vi "singin.vi"(0 "sim I/O info in":T1, 9 "data from node input terminals":variant[](array[variant]), 11 "input from node terminal error in":errorcluster) -> (4 "sim I/O info out":T1, 10 "data to node output terminals":variant[](array[variant]), 15 "output to node terminal error out":errorcluster)   [LabVIEW 2012]
uses:
  <vilib>/FPGA/viExecutionOnDevComputer/simIO/customVI/Sim IO Info.ctl
  <vilib>/rvi/customViForEmulation/niLvFPGAUserSpecifiedEmulationVISupport.lvclass
  <vilib>/FPGA/viExecutionOnDevComputer/simIO/customVI/niFPGA Simulated IO.lvlib
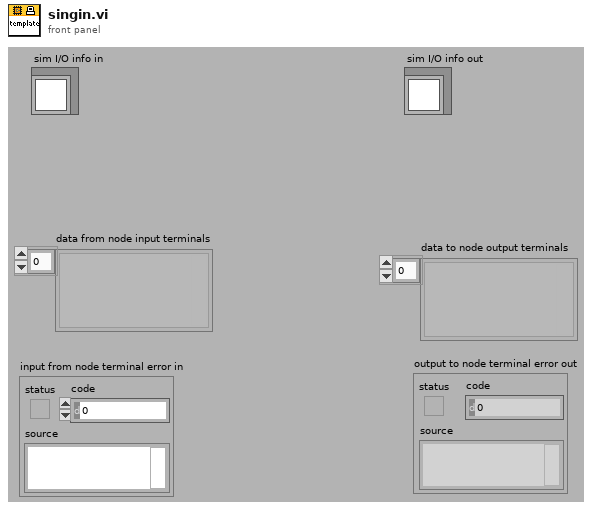
[diagram p1: front panel]
types:
  T1 = typedef "niFPGA Simulated IO.lvlib/Sim IO Info.ctl" = refnum<class "niLvFPGAUserSpecifiedEmulationVISupport.lvclass">
  T2 = typedef "niFPGA Simulated IO.lvlib/Execution Stage.ctl" = enum16{"Initializing", "Running", "Shutting Down"}
  T3 = typedef "niFPGA Simulated IO.lvlib/Node or Element Type.ctl" = enum16{"Read I/O", "Write I/O", "Method", "Read Property", "Write Property"}
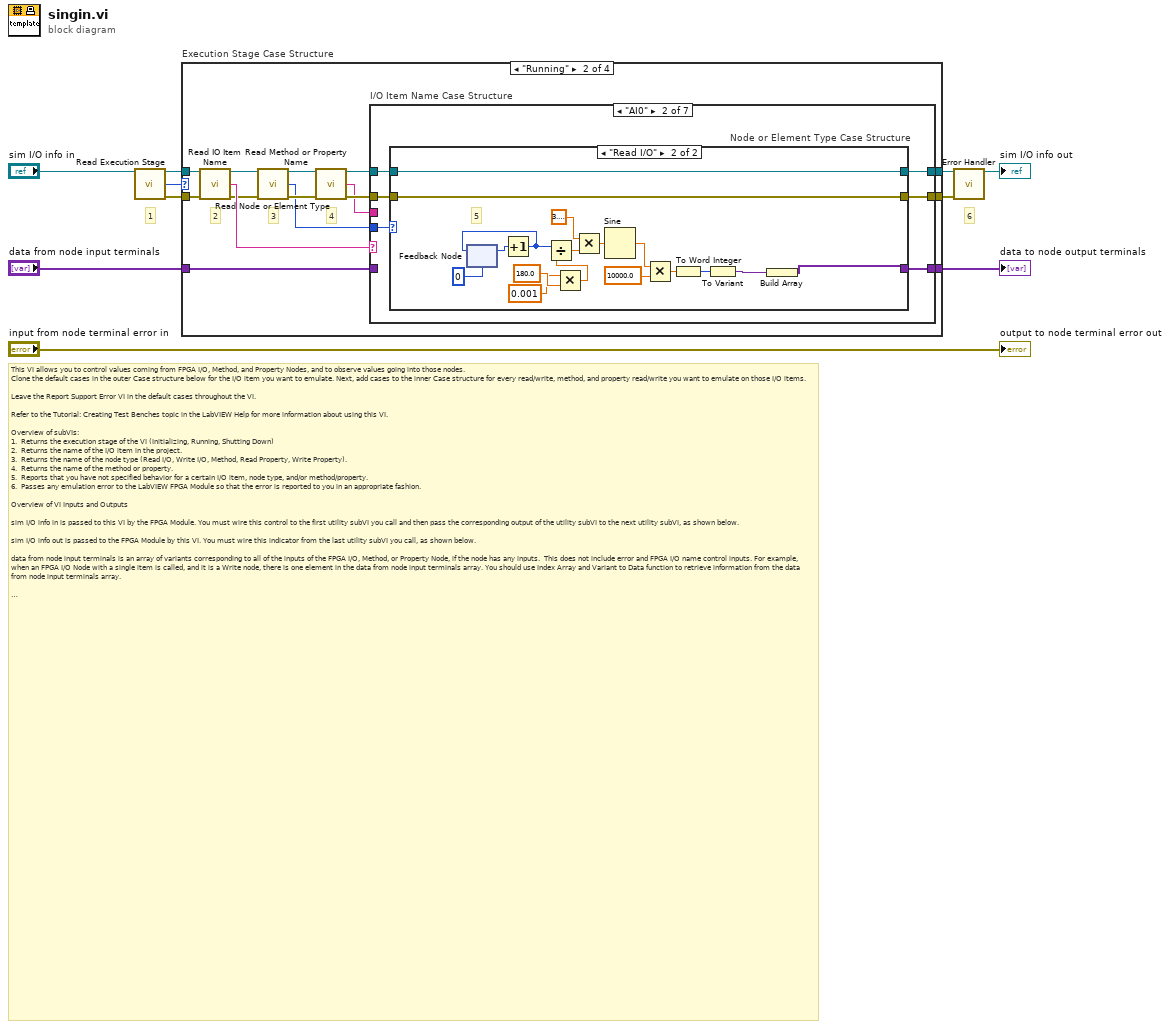
[diagram p0: block diagram]
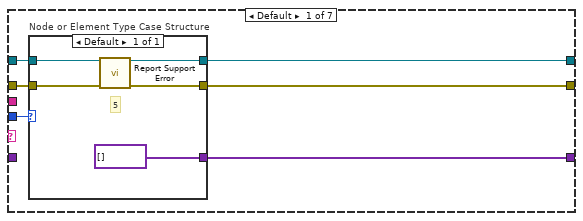
[diagram p3: hidden frame]
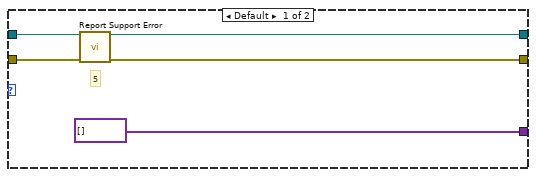
[diagram p4: hidden frame]
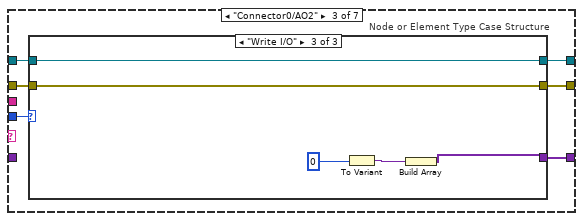
[diagram p5: hidden frame]
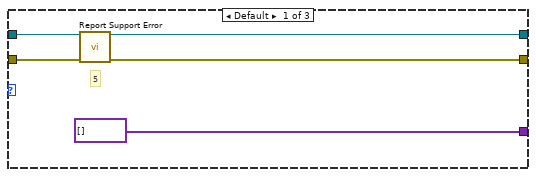
[diagram p6: hidden frame]
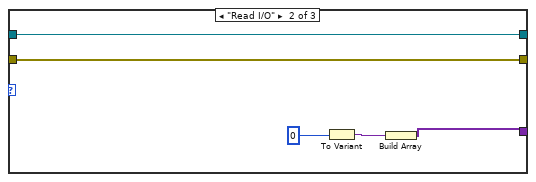
[diagram p7: hidden frame]
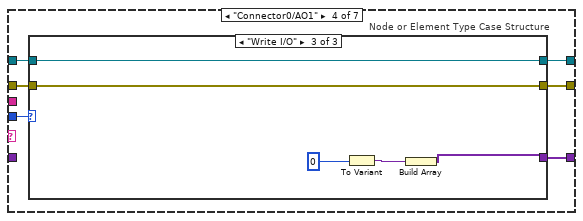
[diagram p8: hidden frame]
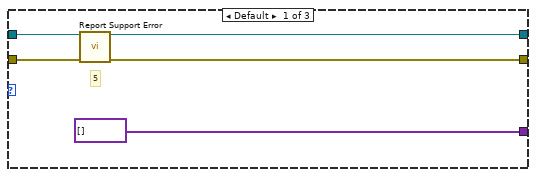
[diagram p9: hidden frame]
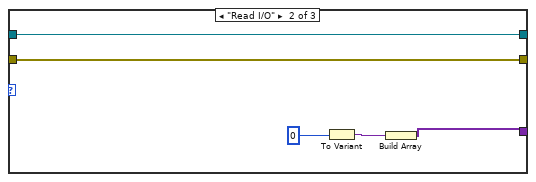
[diagram p10: hidden frame]
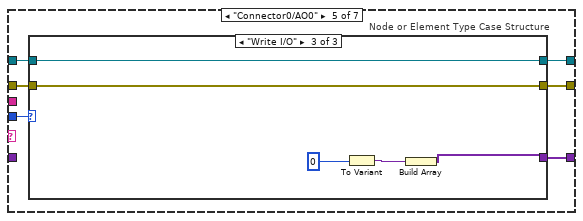
[diagram p11: hidden frame]
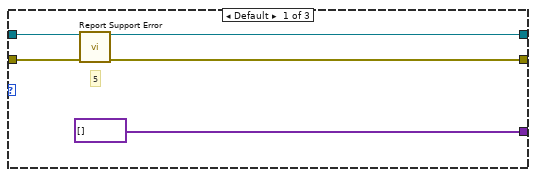
[diagram p12: hidden frame]
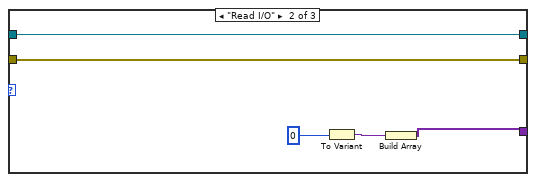
[diagram p13: hidden frame]
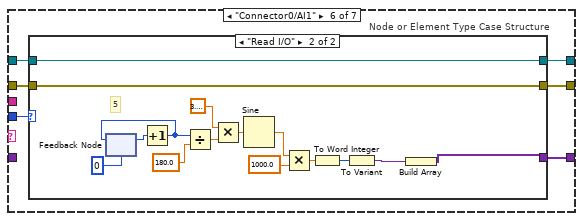
[diagram p14: hidden frame]
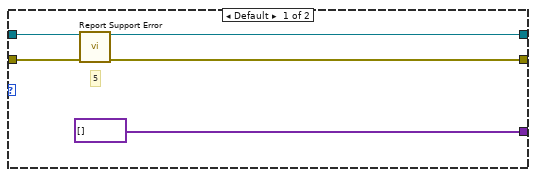
[diagram p15: hidden frame]
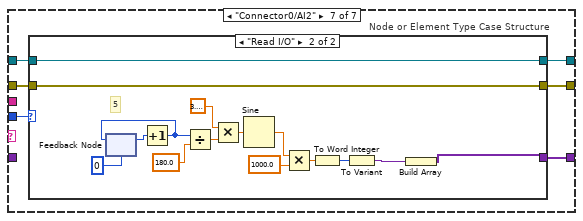
[diagram p16: hidden frame]
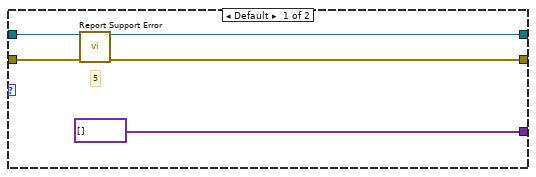
[diagram p17: hidden frame]
diagram:
  # "1"
  # "6"
  # "This VI allows you to control values coming from FPGA I/O, Method, and Property Nodes, and to observe values going into those nodes.\nClone the default cases in the outer Case structure below for the I/O item you want to emulate. Next, add cases to the inner Case structure for every read/write, method, and property read/write you want to emulate on those I/O items.  \n\nLeave the Report Support Error VI in the default cases throughout the VI.\n\nRefer to the Tutorial: Creating Test Benches topic in the LabVIEW Help for more information about using this VI.\n\nOverview of subVIs:\n1.  Returns the execution stage of the VI (Initializing, Running, Shutting Down)\n2.  Returns the name of the I/O item in the project.\n3.  Returns the name of the node type (Read I/O, Write I/O, Method, Read Property, Write Property).\n4.  Returns the name of the method or property.\n5.  Reports that you have not specified behavior for a certain I/O item, node type, and/or method/property.\n6.  Passes any emulation error to the LabVIEW FPGA Module so that the error is reported to you in an appropriate fashion.\n\nOverview of VI Inputs and Outputs\n\nsim I/O info in is passed to this VI by the FPGA Module. You must wire this control to the first utility subVI you call and then pass the corresponding output of the utility subVI to the next utility subVI, as shown below.\n\nsim I/O info out is passed to the FPGA Module by this VI. You must wire this indicator from the last utility subVI you call, as shown below.\n\ndata from node input terminals is an array of variants corresponding to all of the inputs of the FPGA I/O, Method, or Property Node, if the node has any inputs.  This does not include error and FPGA I/O name control inputs. For example, when an FPGA I/O Node with a single item is called, and it is a Write node, there is one element in the data from node input terminals array. You should use Index Array and Variant to Data function to retrieve information from the data from node input terminals array.\n\ndata to node output terminals is an array of variants corresponding to all the outputs of the FPGA I/O, Method, or Property Node, if the node has any outputs.  This does not include error and FPGA I/O name control outputs. For example, when an FPGA I/O node with a single item is called, and it is a Read node, there should be one element in the data to node output terminals array. You should use To Variant and Build Array functions to pass the information to the data to node output terminals array.\n\ninput from node terminal error in is the error that gets passed into the FPGA I/O, Method, or Property Node, if the node is configured so that the error input is shown. If the node is configured so that the error input is not shown, the value of this input corresponds to \"no error\" (status is false, error code is 0). \n\noutput to node terminal error out is the error that gets passed out of the FPGA I/O, Method, or Property Node, if the node is configured so that the error output is shown.  If the node is configured so that the error output is not shown, the value of this output is ignored."
  n1 = call <vilib>:"Read Execution Stage.vi"("sim I/O info in"="sim I/O info in") -> ("sim I/O info out"=w3:T1, "execution stage"=w1:T2, "error out"=w2:errorcluster)  [unwired: 1 in, 11 out]
  n2 = case "Execution Stage Case Structure" shown="\"Running\"" w1 {
    tunnel: [_ w26 _ _] -> w9
    tunnel: [w12 w21 w183 w185] -> w4
    tunnel: [w11 w17 w182 w184] -> w6
    tunnel: w3 -> [w11 w15 w182 w184]
    tunnel: w2 -> [w12 w14 w183 w185]
    tunnel: "data from node input terminals" -> [_ w27 _ _]
    frame "Initializing" {
    }
    frame "Running" {
      # "4"
      # "3"
      # "2"
      n3 = call <vilib>:"Read IO Item Name.vi"("sim I/O info in"=w15, "error in (no error)"=w14) -> ("sim I/O info out"=w16:T1, "I/O item name"=w25:string, "error out"=w24:errorcluster)  [unwired: 11 out]
      n4 = call <vilib>:"Read Node or Element Type.vi"("sim I/O info in"=w16, "error in (no error)"=w24) -> ("sim I/O info out"=w13:T1, "node or element type"=w22:T3, "error out"=w23:errorcluster)  [unwired: 11 out]
      n5 = call <vilib>:"Read Method or Property Name.vi"("sim I/O info in"=w13, "error in (no error)"=w23) -> ("sim I/O info out"=w19:T1, "method or property name"=w18:string, "error out"=w20:errorcluster)  [unwired: 11 out]
      n6 = case "I/O Item Name Case Structure" shown="\"AI0\"" w25 {
        tunnel: w27 -> [_ _ _ _ _ _ _]
        tunnel: [w29 w40 w68 w89 w110 w131 w157] -> w26
        tunnel: w20 -> [w33 w44 w72 w93 w114 w135 w161]
        tunnel: [w32 w43 w71 w92 w113 w134 w160] -> w21
        tunnel: w19 -> [w31 w42 w70 w91 w112 w133 w159]
        tunnel: [w30 w41 w69 w90 w111 w132 w158] -> w17
        tunnel: w22 -> [w28 w39 w67 w88 w109 w130 w156]
        tunnel: w18 -> [_ _ _ _ _ _ _]
        frame Default {
          n7 = case "Node or Element Type Case Structure" shown="Default" w28 {
            tunnel: w33 -> [w38]
            tunnel: [w37] -> w32
            tunnel: w31 -> [w36]
            tunnel: [w35] -> w30
            tunnel: [variant[] []] -> w29
            frame Default {
              # "5"
              n8 = call <vilib>:"Report Support Error.vi"("sim I/O info in"=w36, "error in (no error)"=w38) -> ("sim I/O info out"=w35:T1, "error out"=w37:errorcluster)  [unwired: 12 out]
            }
          }
        }
        frame "AI0" {
          n9 = case "Node or Element Type Case Structure" shown="\"Read I/O\"" w39 {
            tunnel: w44 -> [w49 w65]
            tunnel: [w48 w65] -> w43
            tunnel: w42 -> [w47 w66]
            tunnel: [w46 w66] -> w41
            tunnel: [variant[] [] w55] -> w40
            frame Default {
              # "5"
              n10 = call <vilib>:"Report Support Error.vi"("sim I/O info in"=w47, "error in (no error)"=w49) -> ("sim I/O info out"=w46:T1, "error out"=w48:errorcluster)  [unwired: 12 out]
            }
            frame "Read I/O" {
              # "5"
              n11 = feedback #1(0) -> (w57:i32)
              n12 = Increment(x=w57) -> (x+1=w56:i32)
              n13 = feedback-in #1(w56) -> ()
              n14 = Multiply(x=0.001, y=180.0) -> (x*y=w50:dbl)
              n15 = Divide(x=w56, y=w50) -> (x/y=w59:dbl)
              n16 = Multiply(x=3.141592653589793, y=w59) -> (x*y=w61:dbl)
              n17 = Sine(x=w61) -> (sin(x)=w63:dbl)
              n18 = Multiply(x=w63, y=10000.0) -> (x*y=w64:dbl)
              n19 = To Word Integer(number=w64) -> (16bit integer=w54:i16)
              n20 = To Variant(anything=w54) -> (Variant=w53:variant)
              n21 = Build Array(w53) -> (w55:variant[])
            }
          }
        }
        frame "Connector0/AO2" {
          n22 = case "Node or Element Type Case Structure" shown="\"Write I/O\"" w67 {
            tunnel: w72 -> [w77 w81 w86]
            tunnel: [w76 w81 w86] -> w71
            tunnel: w70 -> [w75 w82 w87]
            tunnel: [w74 w82 w87] -> w69
            tunnel: [variant[] [] w80 w85] -> w68
            frame Default {
              # "5"
              n23 = call <vilib>:"Report Support Error.vi"("sim I/O info in"=w75, "error in (no error)"=w77) -> ("sim I/O info out"=w74:T1, "error out"=w76:errorcluster)  [unwired: 12 out]
            }
            frame "Read I/O" {
              n24 = To Variant(anything=0) -> (Variant=w79:variant)
              n25 = Build Array(w79) -> (w80:variant[])
            }
            frame "Write I/O" {
              n26 = To Variant(anything=0) -> (Variant=w84:variant)
              n27 = Build Array(w84) -> (w85:variant[])
            }
          }
        }
        frame "Connector0/AO1" {
          n28 = case "Node or Element Type Case Structure" shown="\"Write I/O\"" w88 {
            tunnel: w93 -> [w98 w102 w107]
            tunnel: [w97 w102 w107] -> w92
            tunnel: w91 -> [w96 w103 w108]
            tunnel: [w95 w103 w108] -> w90
            tunnel: [variant[] [] w101 w106] -> w89
            frame Default {
              # "5"
              n29 = call <vilib>:"Report Support Error.vi"("sim I/O info in"=w96, "error in (no error)"=w98) -> ("sim I/O info out"=w95:T1, "error out"=w97:errorcluster)  [unwired: 12 out]
            }
            frame "Read I/O" {
              n30 = To Variant(anything=0) -> (Variant=w100:variant)
              n31 = Build Array(w100) -> (w101:variant[])
            }
            frame "Write I/O" {
              n32 = To Variant(anything=0) -> (Variant=w105:variant)
              n33 = Build Array(w105) -> (w106:variant[])
            }
          }
        }
        frame "Connector0/AO0" {
          n34 = case "Node or Element Type Case Structure" shown="\"Write I/O\"" w109 {
            tunnel: w114 -> [w119 w123 w128]
            tunnel: [w118 w123 w128] -> w113
            tunnel: w112 -> [w117 w124 w129]
            tunnel: [w116 w124 w129] -> w111
            tunnel: [variant[] [] w122 w127] -> w110
            frame Default {
              # "5"
              n35 = call <vilib>:"Report Support Error.vi"("sim I/O info in"=w117, "error in (no error)"=w119) -> ("sim I/O info out"=w116:T1, "error out"=w118:errorcluster)  [unwired: 12 out]
            }
            frame "Read I/O" {
              n36 = To Variant(anything=0) -> (Variant=w121:variant)
              n37 = Build Array(w121) -> (w122:variant[])
            }
            frame "Write I/O" {
              n38 = To Variant(anything=0) -> (Variant=w126:variant)
              n39 = Build Array(w126) -> (w127:variant[])
            }
          }
        }
        frame "Connector0/AI1" {
          n40 = case "Node or Element Type Case Structure" shown="\"Read I/O\"" w130 {
            tunnel: w135 -> [w140 w154]
            tunnel: [w139 w154] -> w134
            tunnel: w133 -> [w138 w155]
            tunnel: [w137 w155] -> w132
            tunnel: [variant[] [] w143] -> w131
            frame Default {
              # "5"
              n41 = call <vilib>:"Report Support Error.vi"("sim I/O info in"=w138, "error in (no error)"=w140) -> ("sim I/O info out"=w137:T1, "error out"=w139:errorcluster)  [unwired: 12 out]
            }
            frame "Read I/O" {
              # "5"
              n42 = feedback #2(0) -> (w145:i32)
              n43 = Increment(x=w145) -> (x+1=w144:i32)
              n44 = feedback-in #2(w144) -> ()
              n45 = Divide(x=w144, y=180.0) -> (x/y=w148:dbl)
              n46 = Multiply(x=3.141592653589793, y=w148) -> (x*y=w150:dbl)
              n47 = Sine(x=w150) -> (sin(x)=w152:dbl)
              n48 = Multiply(x=w152, y=1000.0) -> (x*y=w153:dbl)
              n49 = To Word Integer(number=w153) -> (16bit integer=w142:i16)
              n50 = To Variant(anything=w142) -> (Variant=w141:variant)
              n51 = Build Array(w141) -> (w143:variant[])
            }
          }
        }
        frame "Connector0/AI2" {
          n52 = case "Node or Element Type Case Structure" shown="\"Read I/O\"" w156 {
            tunnel: w161 -> [w166 w180]
            tunnel: [w165 w180] -> w160
            tunnel: w159 -> [w164 w181]
            tunnel: [w163 w181] -> w158
            tunnel: [variant[] [] w169] -> w157
            frame Default {
              # "5"
              n53 = call <vilib>:"Report Support Error.vi"("sim I/O info in"=w164, "error in (no error)"=w166) -> ("sim I/O info out"=w163:T1, "error out"=w165:errorcluster)  [unwired: 12 out]
            }
            frame "Read I/O" {
              # "5"
              n54 = feedback #3(0) -> (w171:i32)
              n55 = Increment(x=w171) -> (x+1=w170:i32)
              n56 = feedback-in #3(w170) -> ()
              n57 = Divide(x=w170, y=180.0) -> (x/y=w174:dbl)
              n58 = Multiply(x=3.141592653589793, y=w174) -> (x*y=w176:dbl)
              n59 = Sine(x=w176) -> (sin(x)=w178:dbl)
              n60 = Multiply(x=w178, y=1000.0) -> (x*y=w179:dbl)
              n61 = To Word Integer(number=w179) -> (16bit integer=w168:i16)
              n62 = To Variant(anything=w168) -> (Variant=w167:variant)
              n63 = Build Array(w167) -> (w169:variant[])
            }
          }
        }
      }
    }
    frame "Shutting Down" {
    }
    frame Default {
    }
  }
  "data to node output terminals" <- w9
  n64 = call <vilib>:"Error Handler.vi"("sim I/O info in"=w6, "error in"=w4) -> ("sim I/O info out"=→"sim I/O info out":T1)  [unwired: 13 out]
  "output to node terminal error out" <- "input from node terminal error in"
